vi "View Reports.vi"() -> ()   [LabVIEW 2019, in "View Reports.lvlib"]
uses:
  View Reports.lvlib
  support/States.ctl
  support/StateData.ctl
  <vilib>/Utility/sysdir.llb/System Directory Type.ctl
  <vilib>/Utility/miscctls.llb/LVRowAndColumnTypeDef.ctl
  <vilib>/Utility/file.llb/Read Delimited Spreadsheet (string).vi
panel:
  in  "Open Reports Folder":bool
  in  "Refresh Button":bool
  out "Report Results":string[][](table)
  in  "Reports":i32(listbox)=-1
  # "View Reports"
  # "asdfadsfsfd"
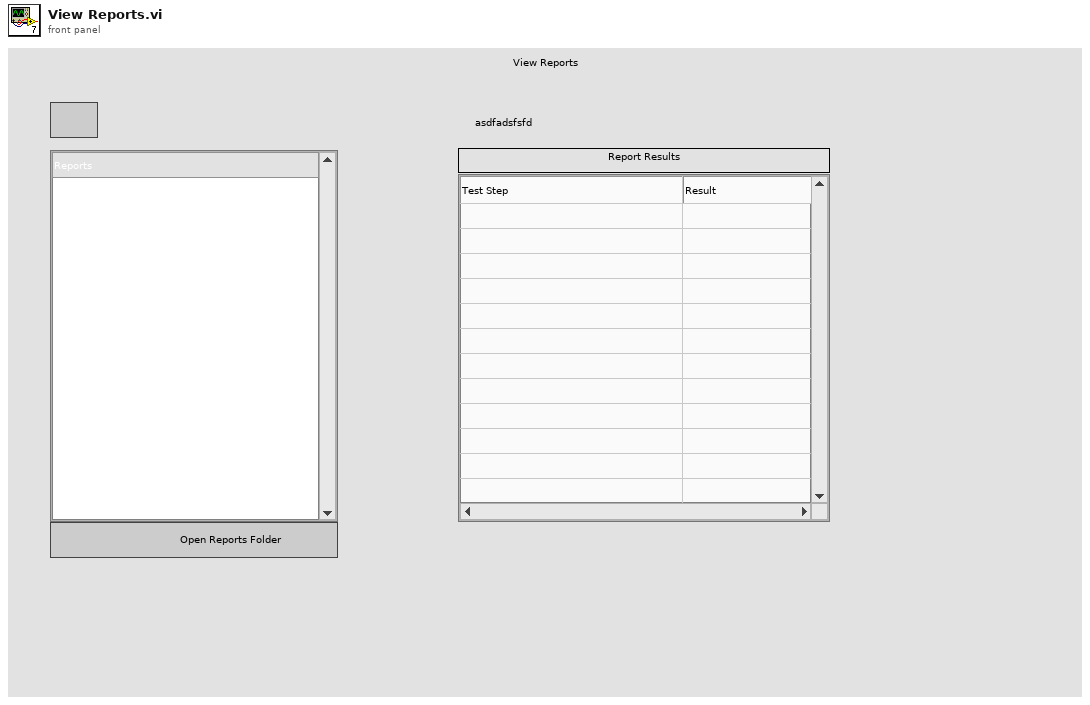
[diagram p1: front panel]
types:
  T1 = typedef "View Reports.lvlib/StateData.ctl" = cluster{"Report filepaths":path[], "Report table":string[][], "Report name":string, "Report folderpath":path}
  T2 = typedef "View Reports.lvlib/States.ctl" = enum16{"Initialize", "Wait for Event", "Refresh Reports List", "Shutdown"}
  T3 = typedef "LVRowAndColumnTypeDef.ctl" = cluster{"Row":i32, "Column":i32}
  T4 = typedef "System Directory Type.ctl" = i32
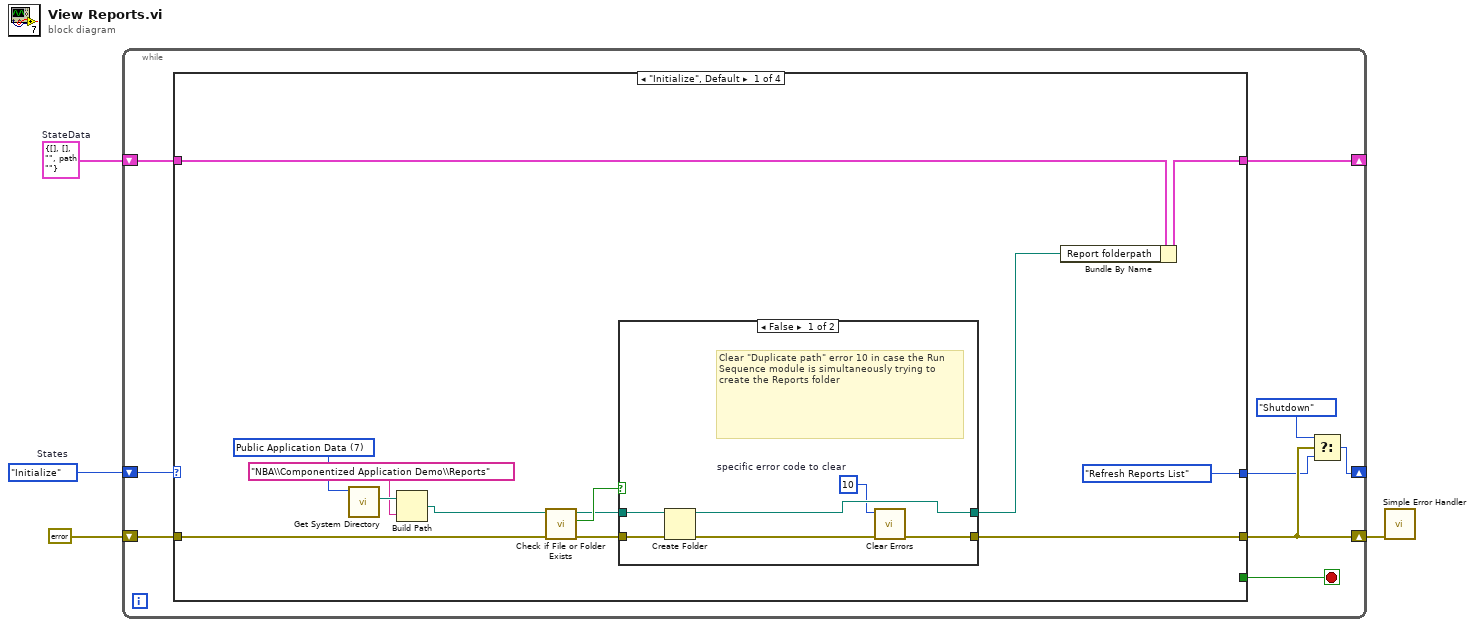
[diagram p0: block diagram]
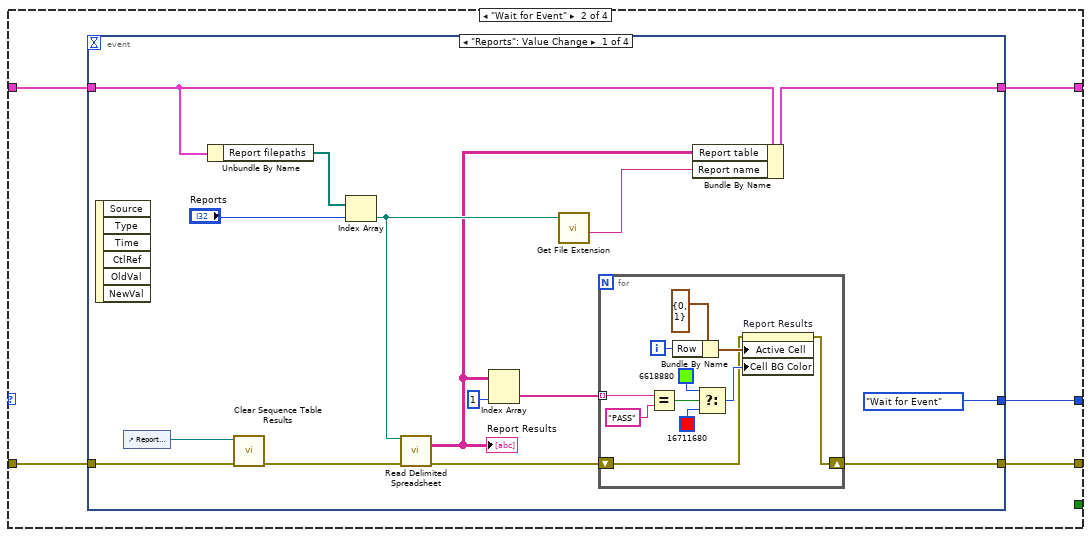
[diagram p3: hidden frame]
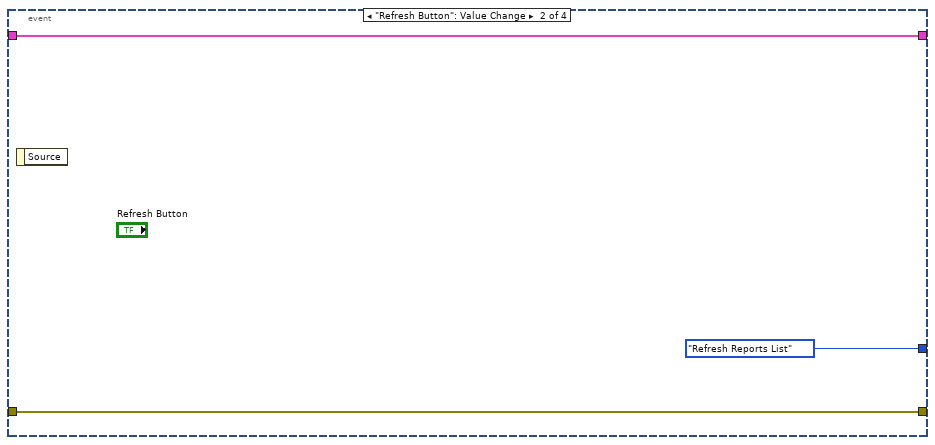
[diagram p4: hidden frame]
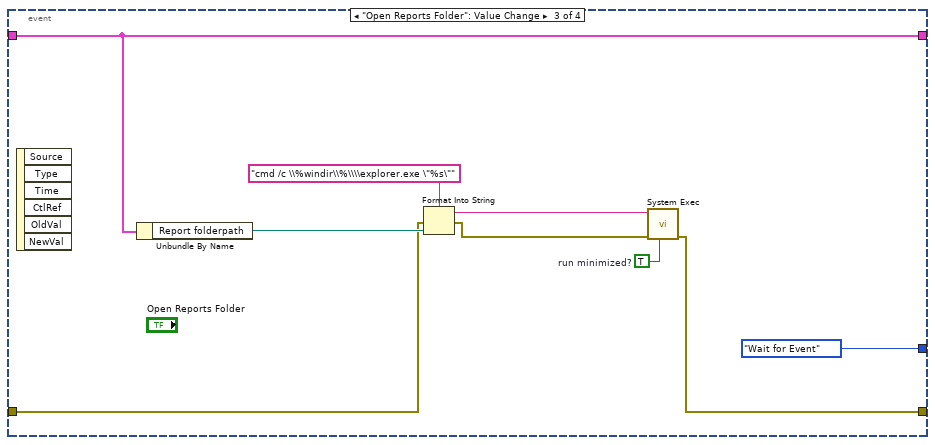
[diagram p5: hidden frame]
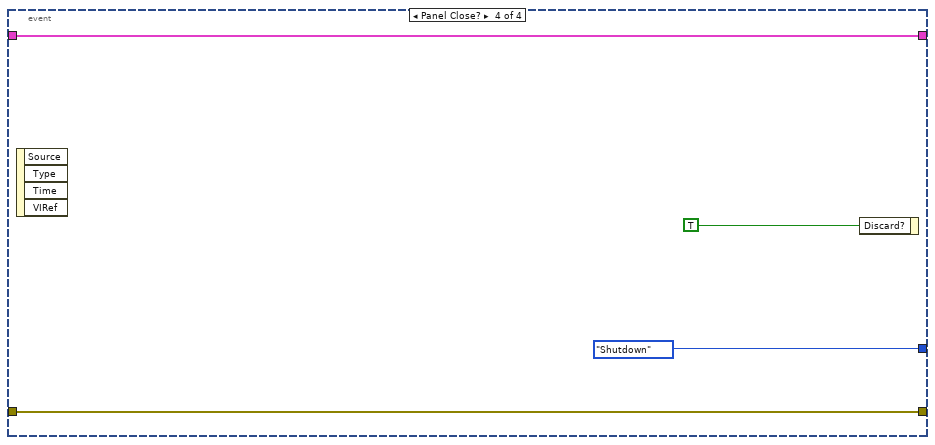
[diagram p6: hidden frame]
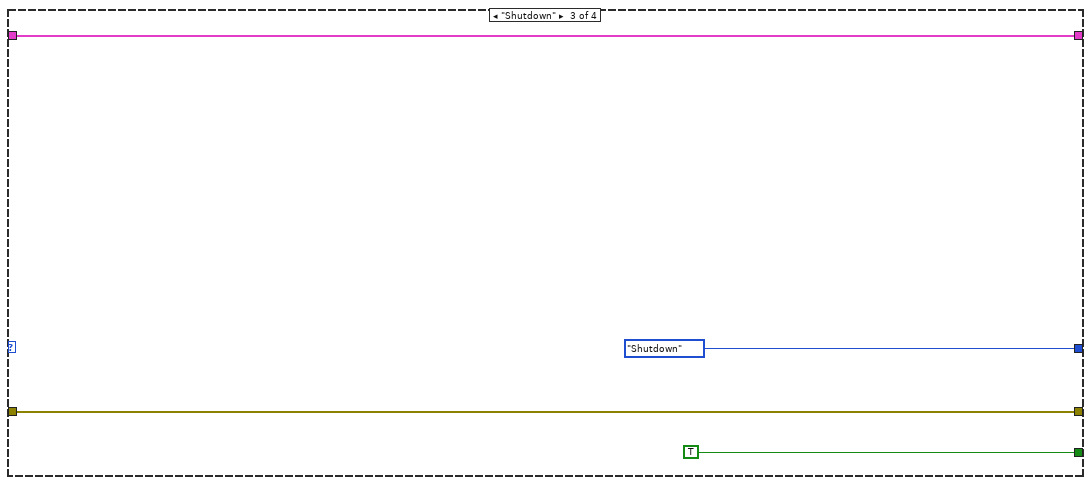
[diagram p7: hidden frame]
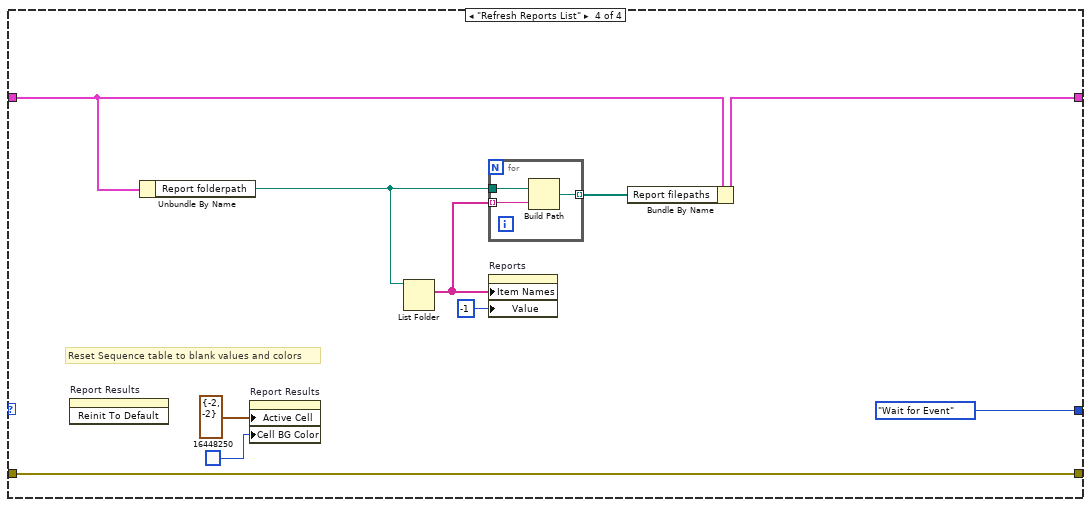
[diagram p8: hidden frame]
diagram:
  w1 = T1 {"Report filepaths"=[], "Report table"=[], "Report name"="", "Report folderpath"=path ""}  # StateData
  w2 = States."Initialize"  # States
  n1 = while {
    shift-right: [w6] -> _
    shift-left: w2 -> [w13]
    shift-right: [w11] -> _
    shift-left: w1 -> [w12]
    shift-right: [w8] -> w3
    shift-left: errorcluster {"status"=FALSE, "code"=0, "source"=""} ("error in (no error)") -> [w9]
    stop <- w10 stop-if-true
    n2 = case shown="\"Initialize\", Default" w13 {
      tunnel: [States."Refresh Reports List" ("ViewReports_States") w39 States."Shutdown" ("ViewReports_States") States."Wait for Event" ("ViewReports_States")] -> w7
      tunnel: w12 -> [w25 w38 w85 w87]
      tunnel: [w15 w37 w85 w92] -> w11
      tunnel: [_ _ TRUE _] -> w10
      tunnel: w9 -> [w20 w36 w83 w95]
      tunnel: [w16 w35 w83 w95] -> w8
      frame "Initialize", Default {
        w24 = T4 7 items=["User Home"=0, "User Desktop"=1, "User Documents"=2, "User Application Data"=3, "User Preferences"=4, "User Temporary"=5, "Public Documents"=6, "Public Application Data"=7, "Public Preferences"=8, "Public Cache"=13, "System Core Libraries"=9, "System Installed Libraries"=10, "Application Files"=11, "Boot Volume Root"=12] ("system directory type")
        n3 = call <vilib>:"Get System Directory.vi"("system directory type"=w24) -> ("system directory"=w23:path)  [unwired: 10 in]
        n4 = Build Path(base path=w23, name or relative path="NBA\\Componentized Application Demo\\Reports") -> (appended path=w21:path)
        n5 = call <vilib>:"Check if File or Folder Exists.vi"("error in (no error)"=w20, "path"=w21) -> ("error out"=w19:errorcluster, "file or folder exists?"=w18:bool, "dup path"=w17:path)  [unwired: 7 in]
        n6 = case shown="False" w18 {
          tunnel: w19 -> [w32 w34]
          tunnel: w17 -> [w31 w33]
          tunnel: [w27 w34] -> w16
          tunnel: [w30 w33] -> w14
          frame False {
            w29 = 10  # specific error code to clear
            # "Clear \"Duplicate path\" error 10 in case the Run Sequence module is simultaneously trying to create the Reports folder"
            n7 = Create Folder(path (use dialog)=w31, error in=w32) -> (created path=w30:path, error out=w28:errorcluster)  [unwired: 1 in, 1 out]
            n8 = call <vilib>:"Clear Errors.vi"("error in (no error)"=w28, "specific error code to clear (0: all)"=w29) -> ("error out"=w27:errorcluster)  [unwired: 4 in, 1 out]
          }
          frame True {
          }
        }
        n9 = Bundle By Name(cluster=w25, "Report folderpath"=w14) -> (w15:T1)
      }
      frame "Wait for Event" {
        n10 = event shown="[0] \"Reports\": Value Change" {
          selector: _ -> [_ _ _ _]
          dyn-events: _ -> [_ _ _ _]
          timeout: _ -> [_ _ _ _]
          tunnel: [States."Wait for Event" ("ViewReports_States") States."Refresh Reports List" ("ViewReports_States") States."Wait for Event" ("ViewReports_States") States."Shutdown" ("ViewReports_States")] -> w39
          tunnel: w38 -> [w54 w68 w74 w80]
          tunnel: [w51 w68 w74 w80] -> w37
          tunnel: w36 -> [w42 w67 w71 w79]
          tunnel: [w43 w67 w70 w79] -> w35
          event "Reports": Value Change {
            n11 = event-data() -> ()  [unwired: 1 in, 6 out]
            n12 = control-ref of="Report Results"() -> (w40:refnum<vi>)
            n13 = Unbundle By Name(w54) -> ("Report filepaths"=w53:path[])
            n14 = call "Clear Sequence Table Results.vi"("error in (no error)"=w42, "table reference in"=w40) -> ("error out"=w41:errorcluster)  [unwired: 8 in, 1 out]
            n15 = Index Array(array=w53, index="Reports") -> (element=w50:path)
            n16 = call-poly <vilib>:"Read Delimited Spreadsheet.vi"("file path (dialog if empty)"=w50, "error in (no error)"=w41) -> ("all rows"=w47:string[][], "error out"=w44:errorcluster)  [unwired: 8 in, 4 out]
            "Report Results" <- w47
            n17 = Index Array(array=w47, index (col)=1 ("disabled index (col)")) -> (element=w45:string[])  [unwired: 1 in]
            n18 = call <vilib>:"Get File Extension.vi"("file"=w50) -> ("filename without extension"=w49:string)  [unwired: 6 in, 4 out]
            n19 = for {
              tunnel: w45 -> [w62] mode=indexing
              shift-right: [w55] -> w43
              shift-left: w44 -> [w56]
              i -> [w63]
              n20 = Equal?(x=w62, y="PASS") -> (x = y?=w60:bool)
              n21 = Bundle By Name(cluster=T3 {"Row"=0, "Column"=1} ("Active Cell:Active Cell"), "Row"=w63) -> (w65:T3)
              n22 = Select(t=u32 6618880, s=w60, f=u32 16711680) -> (s? t:f=w57:u32)
              n23 = property on="Report Results" class="Tbl (strict)"(error in=w56, "Active Cell"=w65, "Cell BG Color"=w57) -> (error out=w55:errorcluster)  [unwired: 1 in, 1 out]
            }
            n24 = Bundle By Name(cluster=w54, "Report table"=w47, "Report name"=w49) -> (w51:T1)
          }
          event "Refresh Button": Value Change {
            n25 = event-data() -> ()  [unwired: 1 in, 1 out]
          }
          event "Open Reports Folder": Value Change {
            w75 = TRUE  # run minimized?
            n26 = event-data() -> ()  [unwired: 1 in, 6 out]
            n27 = Unbundle By Name(w74) -> ("Report folderpath"=w73:path)
            n28 = Format Into String(format string="cmd /c \\%windir\\%\\\\explorer.exe \"%s\"" ("name or relative path"), error in=w71, w73) -> (resulting string=w76:string, error out=w72:errorcluster)  [unwired: 1 in]
            n29 = call <vilib>:"System Exec.vi"("run minimized? (F)"=w75, "error in (no error)"=w72, "command line"=w76) -> ("error out"=w70:errorcluster)  [unwired: 5 in, 3 out]
          }
          event Panel Close? {
            n30 = event-data() -> ()  [unwired: 1 in, 4 out]
            n31 = event-data("Discard?"=TRUE) -> ()  [unwired: 1 in, 1 out]
          }
        }
      }
      frame "Shutdown" {
      }
      frame "Refresh Reports List" {
        # "Reset Sequence table to blank values and colors"
        n32 = invoke on="Report Results" class="Tbl (strict)" method="Reinit To Default"() -> ()  [unwired: 3 in, 3 out]
        n33 = Unbundle By Name(w87) -> ("Report folderpath"=w86:path)
        n34 = property on="Report Results" class="Tbl (strict)"("Active Cell"=T3 {"Row"=-2, "Column"=-2} ("Active Cell:Active Cell"), "Cell BG Color"=u32 16448250) -> ()  [unwired: 2 in, 2 out]
        n35 = List Folder(path=w86) -> (filenames=w94:string[])  [unwired: 3 in, 3 out]
        n36 = for {
          tunnel: w86 -> [w98]
          tunnel: w94 -> [w97] mode=indexing
          tunnel: [w96] -> w91 mode=indexing
          n37 = Build Path(base path=w98, name or relative path=w97) -> (appended path=w96:path)
        }
        n38 = property on="Reports" class="LstBox (strict)"("Item Names"=w94, "Value"=-1 ("Select Sequence")) -> ()  [unwired: 2 in, 2 out]
        n39 = Bundle By Name(cluster=w87, "Report filepaths"=w91) -> (w92:T1)
      }
    }
    n40 = Select(t=States."Shutdown" ("ViewReports_States"), s=w8, f=w7) -> (s? t:f=w6:T2)
  }
  n41 = call <vilib>:"Simple Error Handler.vi"("error in (no error)"=w3) -> ()  [unwired: 4 in, 5 out]
